vi "Физ задача другой варик.vi"() -> ()   [LabVIEW 2021]
panel:
  out "Q":T1
  out "Сообщение 2":string
  out "Сообщения об ошибках":string
  in  "Вещество":T2 items=["Лед/вода", "Свинец", "Спирт"]
  in  "Масса":T1
  out "Состояние":T3
  in  "Конечная\n температура":T4
  in  "Начальная\n температура":T5
  # "Нагрев"
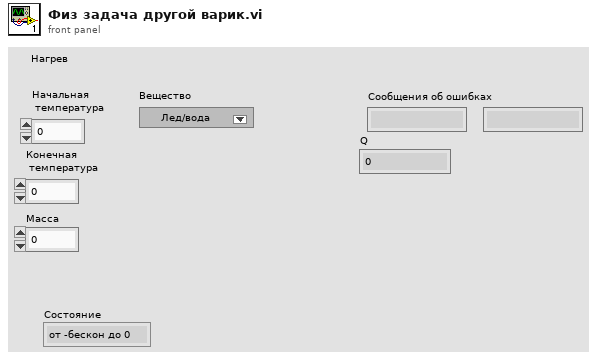
[diagram p1: front panel]
types:
  T1 = typedef "физ5.ctl" = dbl
  T2 = typedef "физ4.ctl" = u16
  T3 = typedef "физ1.ctl" = enum16{"от -бескон до 0", "от 0 до 0", "от 0 до 100", "от 100 до 100", "от 100 до +бескон", "Ошибка"}
  T4 = typedef "физ2.ctl" = dbl
  T5 = typedef "физ3.ctl" = dbl
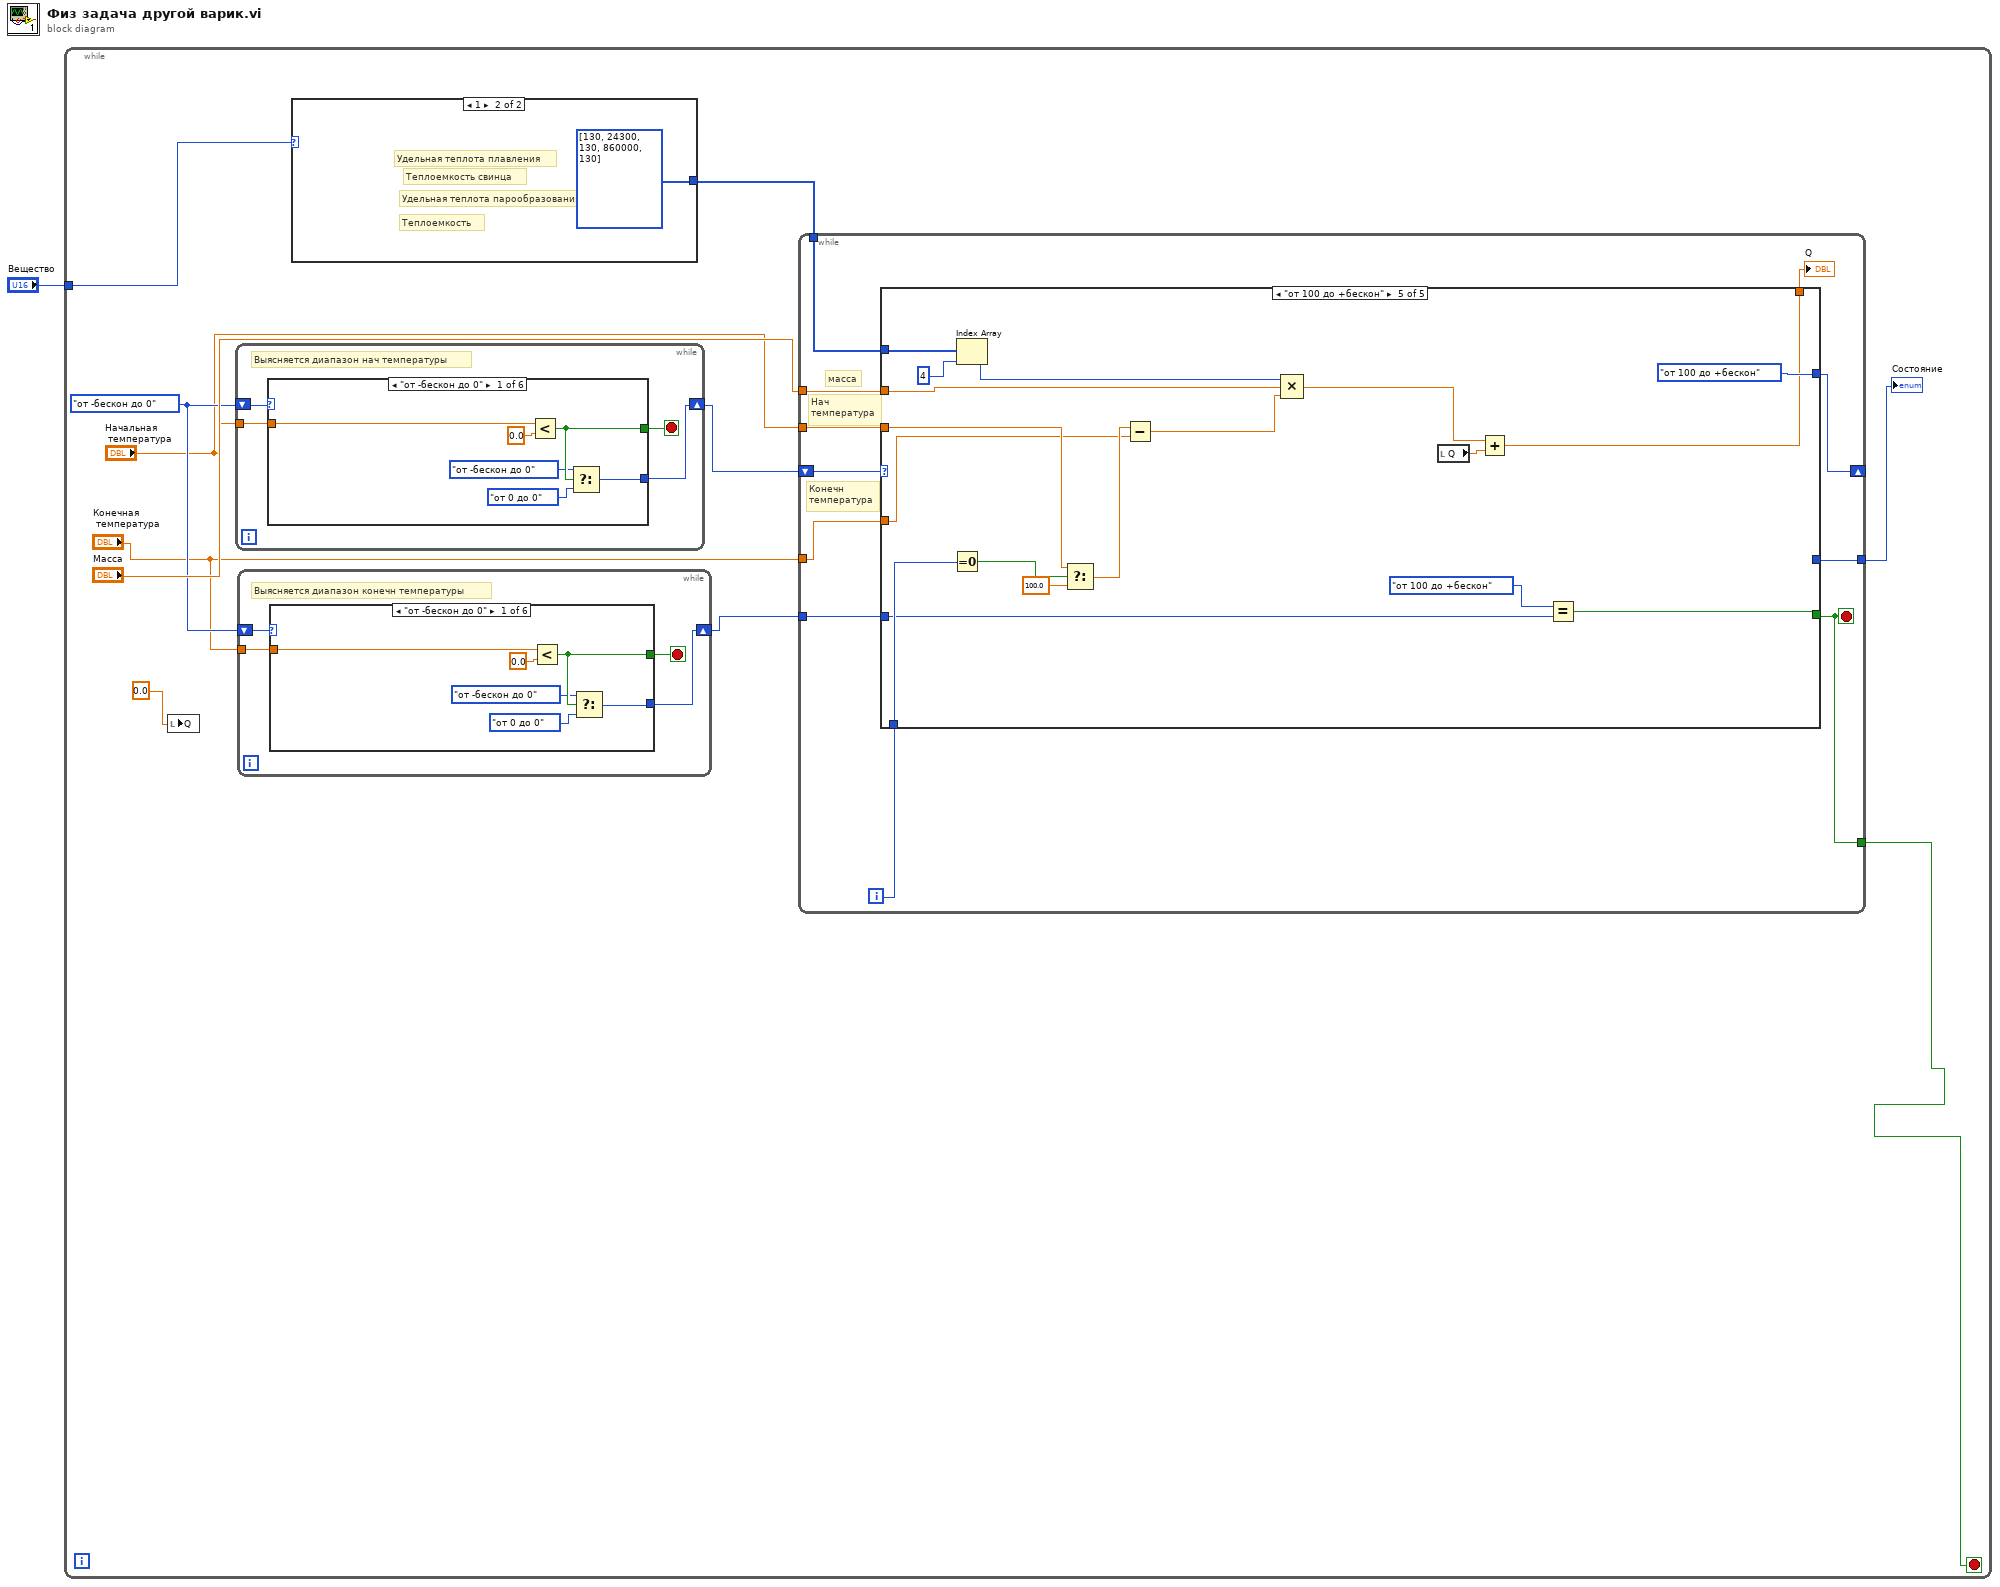
[diagram p0: block diagram]
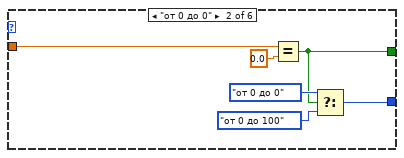
[diagram p2: hidden frame]
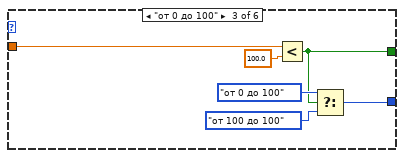
[diagram p3: hidden frame]
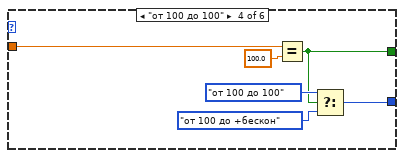
[diagram p4: hidden frame]
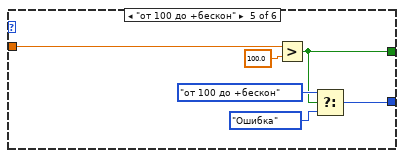
[diagram p5: hidden frame]
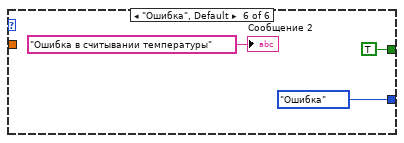
[diagram p6: hidden frame]
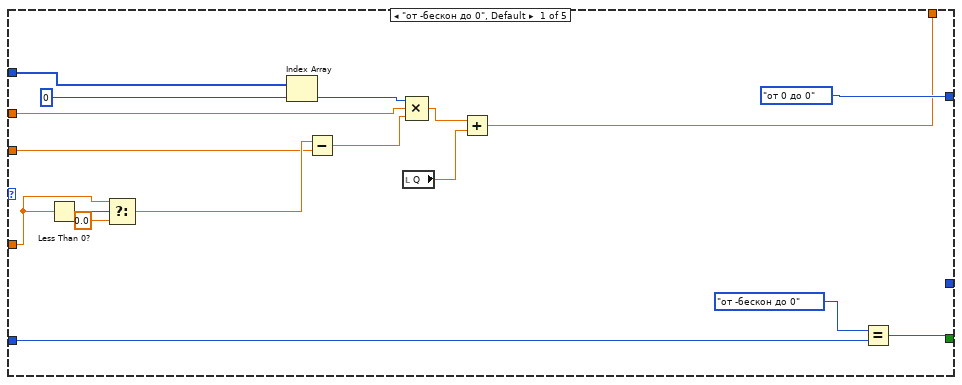
[diagram p7: hidden frame]
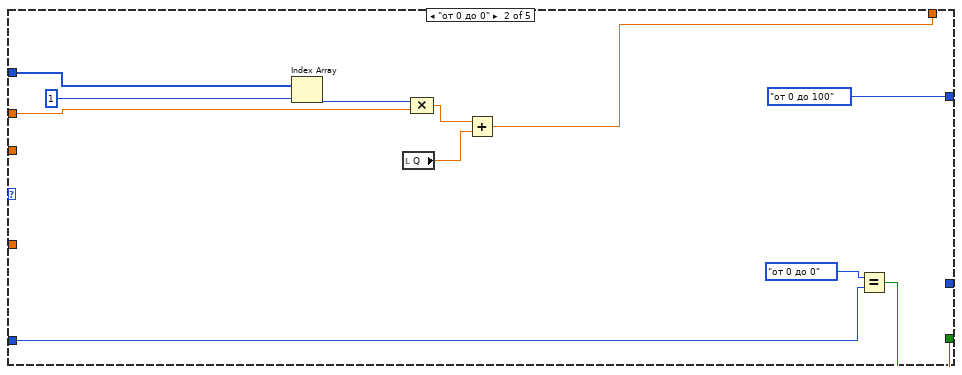
[diagram p8: hidden frame]
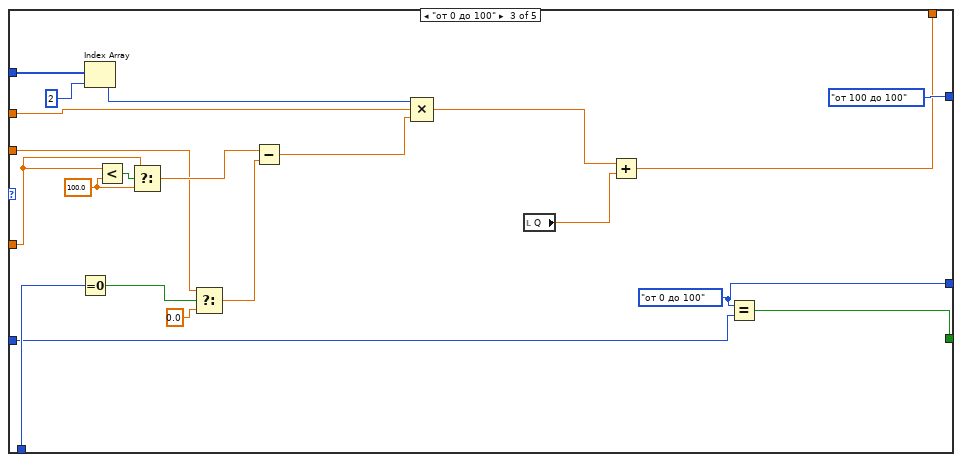
[diagram p9: hidden frame]
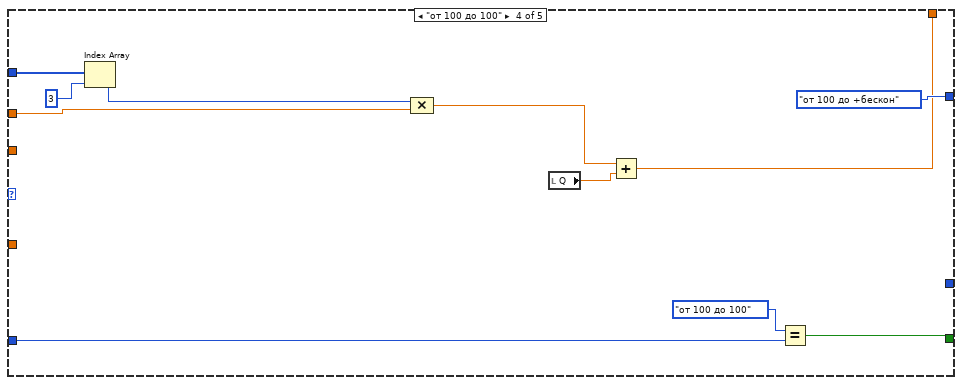
[diagram p10: hidden frame]
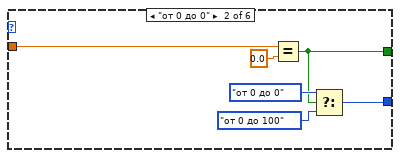
[diagram p11: hidden frame]
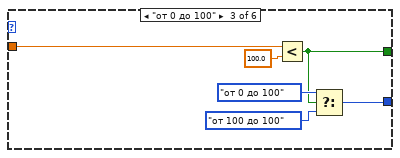
[diagram p12: hidden frame]
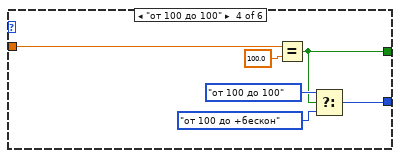
[diagram p13: hidden frame]
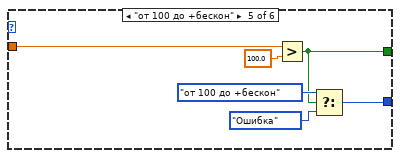
[diagram p14: hidden frame]
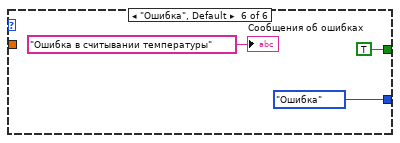
[diagram p15: hidden frame]
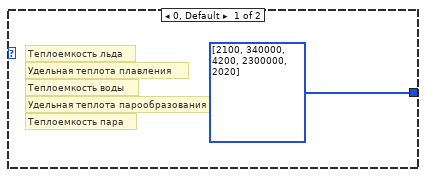
[diagram p16: hidden frame]
diagram:
  n1 = while {
    tunnel: "Вещество" -> [w12]
    stop <- w3 stop-if-true
    w8 = физ1."от -бескон до 0" ("Enum")
    n2 = local write "Q"(T1 0.0 ("x+y")) -> ()
    n3 = while {
      shift-right: [w140] -> w9
      shift-left: w8 -> [w139]
      tunnel: "Начальная\n температура" -> [w142]
      stop <- w141 stop-if-true
      # "Выясняется диапазон нач температуры"
      n4 = case shown="\"от -бескон до 0\"" w139 {
        tunnel: w142 -> [w147 w152 w156 w163 w167 _]
        tunnel: [w144 w150 w157 w162 w170 физ1."Ошибка" ("Enum")] -> w140
        tunnel: [w146 w149 w155 w161 w169 TRUE] -> w141
        frame "от -бескон до 0" {
          n5 = Less?(x=w147, y=T5 0.0) -> (x < y?=w146:bool)
          n6 = Select(t=физ1."от -бескон до 0" ("Enum"), s=w146, f=физ1."от 0 до 0" ("Enum")) -> (s? t:f=w144:T3)
        }
        frame "от 0 до 0" {
          n7 = Equal?(x=w152, y=T5 0.0) -> (x = y?=w149:bool)
          n8 = Select(t=физ1."от 0 до 0" ("Enum"), s=w149, f=физ1."от 0 до 100" ("Enum")) -> (s? t:f=w150:T3)
        }
        frame "от 0 до 100" {
          n9 = Less?(x=w156, y=T5 100.0) -> (x < y?=w155:bool)
          n10 = Select(t=физ1."от 0 до 100" ("Enum"), s=w155, f=физ1."от 100 до 100" ("Enum")) -> (s? t:f=w157:T3)
        }
        frame "от 100 до 100" {
          n11 = Equal?(x=w163, y=T5 100.0) -> (x = y?=w161:bool)
          n12 = Select(t=физ1."от 100 до 100" ("Enum"), s=w161, f=физ1."от 100 до +бескон" ("Enum")) -> (s? t:f=w162:T3)
        }
        frame "от 100 до +бескон" {
          n13 = Greater?(x=w167, y=T5 100.0) -> (0:w169:bool)
          n14 = Select(t=физ1."от 100 до +бескон" ("Enum"), s=w169, f=физ1."Ошибка" ("Enum")) -> (s? t:f=w170:T3)
        }
        frame "Ошибка", Default {
          "Сообщения об ошибках" <- "Ошибка в считывании температуры" ("Сообщение")
        }
      }
    }
    n15 = while {
      shift-right: [w15] -> w5
      shift-left: w8 -> [w14]
      tunnel: "Конечная\n температура" -> [w13]
      stop <- w16 stop-if-true
      # "Выясняется диапазон конечн температуры"
      n16 = case shown="\"от -бескон до 0\"" w14 {
        tunnel: [w19 w25 w31 w37 w44 физ1."Ошибка" ("Enum")] -> w15
        tunnel: [w21 w24 w30 w36 w43 TRUE] -> w16
        tunnel: w13 -> [w17 w23 w29 w35 w41 _]
        frame "от -бескон до 0" {
          n17 = Less?(x=w17, y=T5 0.0) -> (x < y?=w21:bool)
          n18 = Select(t=физ1."от -бескон до 0" ("Enum"), s=w21, f=физ1."от 0 до 0" ("Enum")) -> (s? t:f=w19:T3)
        }
        frame "от 0 до 0" {
          n19 = Equal?(x=w23, y=T5 0.0) -> (x = y?=w24:bool)
          n20 = Select(t=физ1."от 0 до 0" ("Enum"), s=w24, f=физ1."от 0 до 100" ("Enum")) -> (s? t:f=w25:T3)
        }
        frame "от 0 до 100" {
          n21 = Less?(x=w29, y=T5 100.0) -> (x < y?=w30:bool)
          n22 = Select(t=физ1."от 0 до 100" ("Enum"), s=w30, f=физ1."от 100 до 100" ("Enum")) -> (s? t:f=w31:T3)
        }
        frame "от 100 до 100" {
          n23 = Equal?(x=w35, y=T5 100.0) -> (x = y?=w36:bool)
          n24 = Select(t=физ1."от 100 до 100" ("Enum"), s=w36, f=физ1."от 100 до +бескон" ("Enum")) -> (s? t:f=w37:T3)
        }
        frame "от 100 до +бескон" {
          n25 = Greater?(x=w41, y=T5 100.0) -> (0:w43:bool)
          n26 = Select(t=физ1."от 100 до +бескон" ("Enum"), s=w43, f=физ1."Ошибка" ("Enum")) -> (s? t:f=w44:T3)
        }
        frame "Ошибка", Default {
          "Сообщение 2" <- "Ошибка в считывании температуры" ("Сообщение")
        }
      }
    }
    n27 = case shown="1" w12 {
      tunnel: [i32[] [2100, 340000, 4200, 2300000, 2020] i32[] [130, 24300, 130, 860000, 130]] -> w11
      frame 0, Default {
        # "Удельная теплота плавления"
        # "Удельная теплота парообразования"
        # "Теплоемкость пара"
        # "Теплоемкость воды"
        # "Теплоемкость льда"
      }
      frame 1 {
        # "Удельная теплота плавления"
        # "Удельная теплота парообразования"
        # "Теплоемкость"
        # "Теплоемкость свинца"
      }
    }
    n28 = while {
      tunnel: w11 -> [w60]
      tunnel: "Масса" -> [w59]
      tunnel: "Начальная\n температура" -> [w58]
      tunnel: "Конечная\n температура" -> [w57]
      shift-right: [w56] -> _
      shift-left: w9 -> [w55]
      tunnel: w5 -> [w53]
      tunnel: [w51] -> w3
      tunnel: [w50] -> w2
      i -> [w54]
      stop <- w51 stop-if-true
      # "Конечн\nтемпература"
      # "Нач \nтемпература"
      # "масса"
      n29 = case shown="\"от 100 до +бескон\"" w55 {
        tunnel: w60 -> [w77 w86 w107 w118 w136]
        tunnel: w59 -> [w74 w84 w105 w116 w134]
        tunnel: w58 -> [w63 _ w96 _ w128]
        tunnel: w57 -> [w70 _ w102 _ w124]
        tunnel: [физ1."от 0 до 0" ("Enum") физ1."от 0 до 100" ("Enum") физ1."от 100 до 100" ("Enum") физ1."от 100 до +бескон" ("Enum") физ1."от 100 до +бескон" ("Enum")] -> w56
        tunnel: w54 -> [_ _ w99 _ w132]
        tunnel: w53 -> [w67 w81 w92 w113 w126]
        tunnel: [w66 w83 w94 w115 w125] -> w51
        tunnel: [w65 w80 w91 w112 w123] -> w52
        tunnel: [_ _ w89 _ _] -> w50
        frame "от -бескон до 0", Default {
          n30 = Less Than 0?(x=w70) -> (x < 0?=w71:bool)
          n31 = Select(t=w70, s=w71, f=T4 0.0) -> (s? t:f=w64:T4)
          n32 = Index Array(array=w77, index=0) -> (element=w75:i32)
          n33 = Subtract(x=w64, y=w63) -> (x-y=w73:T4)
          n34 = local read "Q"() -> (w62:T1)
          n35 = Compound Arithmetic op=MULTIPLY(w75, w74, w73) -> (w72:T1)
          n36 = Add(x=w72, y=w62) -> (x+y=w65:T1)
          n37 = Equal?(x=физ1."от -бескон до 0" ("Enum"), y=w67) -> (x = y?=w66:bool)
        }
        frame "от 0 до 0" {
          n38 = Index Array(array=w86, index=1) -> (element=w85:i32)
          n39 = local read "Q"() -> (w79:T1)
          n40 = Compound Arithmetic op=MULTIPLY(w85, w84) -> (w87:T1)
          n41 = Add(x=w87, y=w79) -> (x+y=w80:T1)
          n42 = Equal?(x=физ1."от 0 до 0" ("Enum"), y=w81) -> (x = y?=w83:bool)
        }
        frame "от 0 до 100" {
          w89 = физ1."от 0 до 100" ("Enum")
          w103 = T4 100.0 ("f")
          n43 = Equal To 0?(x=w99) -> (x = 0?=w97:bool)
          n44 = Index Array(array=w107, index=2) -> (element=w106:i32)
          n45 = Less?(x=w102, y=w103) -> (x < y?=w104:bool)
          n46 = Select(t=w102, s=w104, f=w103) -> (s? t:f=w101:T4)
          n47 = Select(t=w96, s=w97, f=T4 0.0) -> (s? t:f=w95:T4)
          n48 = Subtract(x=w101, y=w95) -> (x-y=w100:T4)
          n49 = Compound Arithmetic op=MULTIPLY(w106, w105, w100) -> (w108:T1)
          n50 = local read "Q"() -> (w90:T1)
          n51 = Add(x=w108, y=w90) -> (x+y=w91:T1)
          n52 = Equal?(x=w89, y=w92) -> (x = y?=w94:bool)
        }
        frame "от 100 до 100" {
          n53 = Index Array(array=w118, index=3) -> (element=w117:i32)
          n54 = Compound Arithmetic op=MULTIPLY(w117, w116) -> (w119:T1)
          n55 = local read "Q"() -> (w111:T1)
          n56 = Add(x=w119, y=w111) -> (x+y=w112:T1)
          n57 = Equal?(x=физ1."от 100 до 100" ("Enum"), y=w113) -> (x = y?=w115:bool)
        }
        frame "от 100 до +бескон" {
          n58 = Equal To 0?(x=w132) -> (x = 0?=w131:bool)
          n59 = Index Array(array=w136, index=4) -> (element=w135:i32)
          n60 = Select(t=w128, s=w131, f=100.0) -> (s? t:f=w130:T5)
          n61 = Subtract(x=w130, y=w124) -> (x-y=w133:T5)
          n62 = Compound Arithmetic op=MULTIPLY(w135, w134, w133) -> (w137:T1)
          n63 = local read "Q"() -> (w122:T1)
          n64 = Add(x=w137, y=w122) -> (x+y=w123:T1)
          n65 = Equal?(x=физ1."от 100 до +бескон" ("Enum"), y=w126) -> (x = y?=w125:bool)
        }
      }
      "Q" <- w52
    }
    "Состояние" <- w2
  }
